vi "Time Delay with Error.vi"(8 "error in (no error)":errorcluster, 10 "Delay Time (s)":dbl=1.0) -> (0 "error out":errorcluster)   [LabVIEW 2024]
doc: "Inserts a time delay into the calling VI."
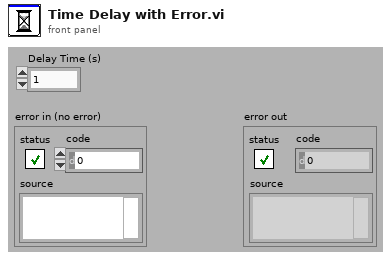
[diagram p1: front panel]
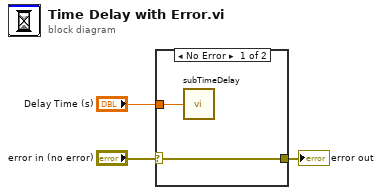
[diagram p0: block diagram]
diagram:
  n1 = case shown="No Error" "error in (no error)" {
    selector: "error in (no error)" -> [w4 w6]
    tunnel: "Delay Time (s)" -> [w5 _]
    tunnel: [w4 w6] -> w1
    frame No Error {
      n2 = call <vilib>:"subTimeDelay.vi"("Delay Time (Seconds)"=w5) -> ()
    }
    frame Error {
    }
  }
  "error out" <- w1
